vi "UserInterface.vi"() -> ()   [LabVIEW 2018]
panel:
  in  "Tab Control":T1(tab)
  in  "CISCO Stats":string(tree)
  in  "Stop":bool
  in  "Refresh":bool
  in  "Configure Mapping":bool
  in  "Report Settings":bool
  in  "Refresh":bool
  in  "Clear Folder":bool
  in  "Cancel Request":bool
  in  "Request Report":bool
  out "Mapped AEs":i32(listbox)
  in  "New AEs":string(combo)
  out "Report Available":bool
  out "Available weeks":string
  out "Request ID":string
  out "Update Required?":bool=TRUE
  in  "Available Reports":i32(listbox)
  in  "Display Stats":bool
  out "Data Display":T2(array[cluster]) {"Open SRs" scale=0.0..40.0; "Solved in more then 5 Workdays" scale=0.0..40.0; "In Work SRs" scale=0.0..40.0; "Solved Within 5 workdays" scale=0.0..40.0; "New SRs" scale=0.0..40.0}
  in  "Year":i16=1 min=1904 max=2019 step=1
  in  "Week":i16=1 min=1 max=52 step=1
  out "Open SRs":u32(colorbox)=16711680
  out "Solved in more then 5 workdays":u32(colorbox)=16753962
  out "In work":u32(colorbox)=9567230
  out "Solved within 5 workdays":u32(colorbox)=6618880
  out "New SRs":u32(colorbox)=16860
  in  "Save to File":bool
  in  "Filters Configuration":bool
  in  "View Selection":T3(ring)
  in  "SRs Queue":string(tree)
  out "End Date":timestamp format="%<%x>T"
  out "Start Date":timestamp format="%<%x>T"
  in  "SR Linkage":string[][](table)
  in  "AE Stats":string[][](table)
  in  "KCS Linkage":bool
  in  "Filters Configuration 2":bool
  in  "AE Selection":enum16{""}(ring)
  in  "SRs View":string(tree)
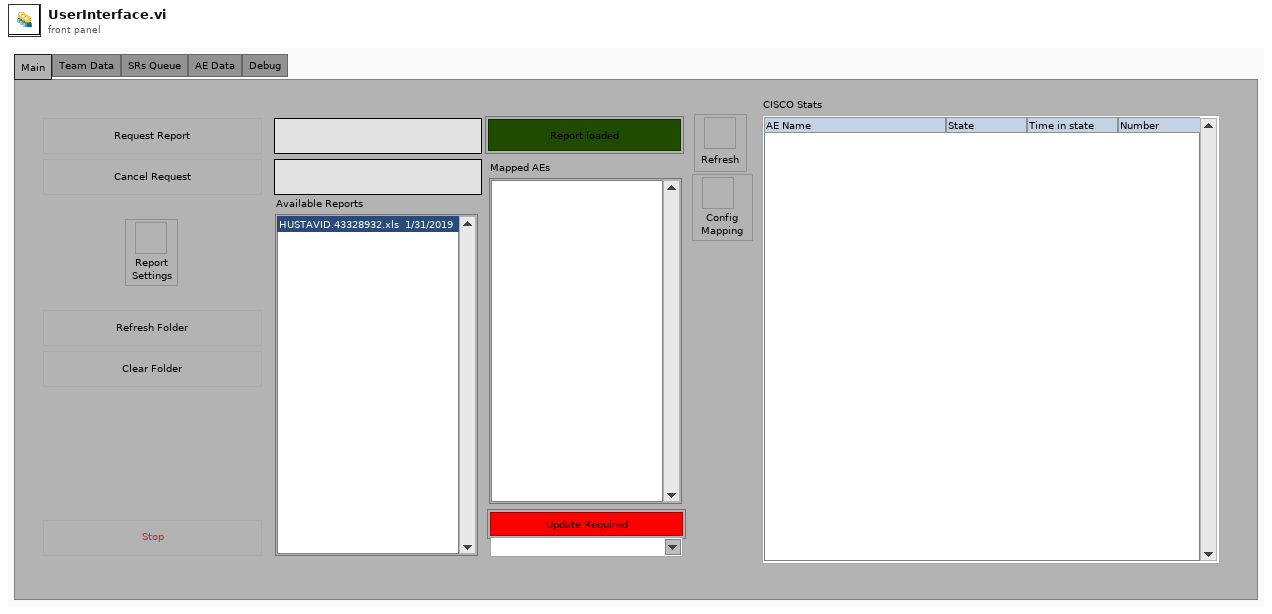
[diagram p1: front panel]
types:
  T1 = enum32{"Main", "Team Data", "SRs Queue", "AE Data", "Debug"}
  T2 = cluster{"New SRs":u8, "Solved Within 5 workdays":u8, "In Work SRs":u8, "Solved in more then 5 Workdays":u8, "Open SRs":u8, "AE-Team":string}[]
  T3 = enum16{"Open", "In Work", "View All", "Neglected"}
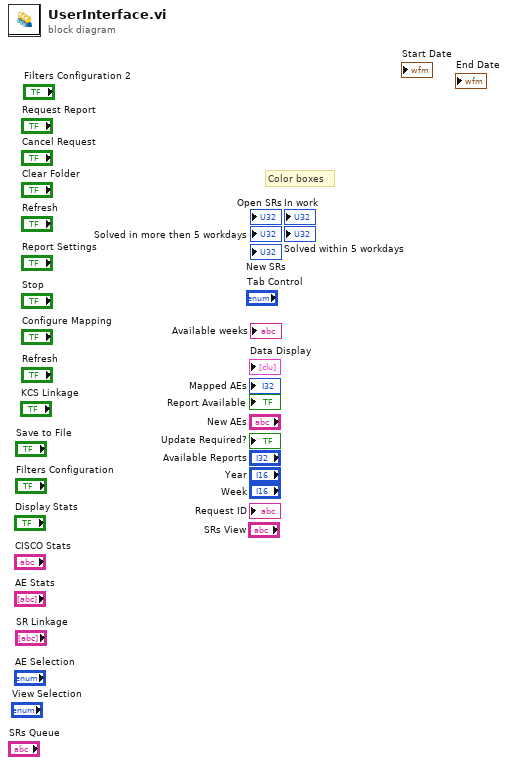
[diagram p0: block diagram]
diagram:
  # "Color boxes"
